vi "test Import To Empty Module Different Slot.vi"(8 "error in (no error)":errorcluster, 11 "TestCase in":refnum<class "SLSC Switch Import Export Unit Tests.lvclass">) -> (0 "error out":errorcluster, 3 "TestCase out":refnum<class "SLSC Switch Import Export Unit Tests.lvclass">)   [LabVIEW 2017, in "SLSC Switch Import Export Unit Tests.lvclass"]
uses:
  SLSC Switch Import Export Unit Tests.lvclass
  Shared/Endpoint Configuration Cluster.ctl
  Shared/Endpoint Configuration Enum.ctl
  SLSC Switch Import Export Unit Tests.lvclass/SLSC Switch Import Export Unit Tests.ctl
  <vilib>/NI Veristand/Custom Device API/Get Item Property (U32).vi
  <vilib>/addons/_JKI Toolkits/VI Tester/TestCase.llb/TestCase.lvclass
  <vilib>/NI/NI VeriStand Custom Device Import and Export Tool/ImportExport.lvlib
  Scripting/SLSC Switch Scripting.lvlib
  Shared/SLSC Switch Shared.lvlib
  <vilib>/NI VeriStand/Custom Device API/Custom Device API.lvlib
  C:/Program Files (x86)/National Instruments/LabVIEW 2017/vi.lib/addons/_JKI Toolkits/VI Tester/TestCase.llb/TestCase.lvclass
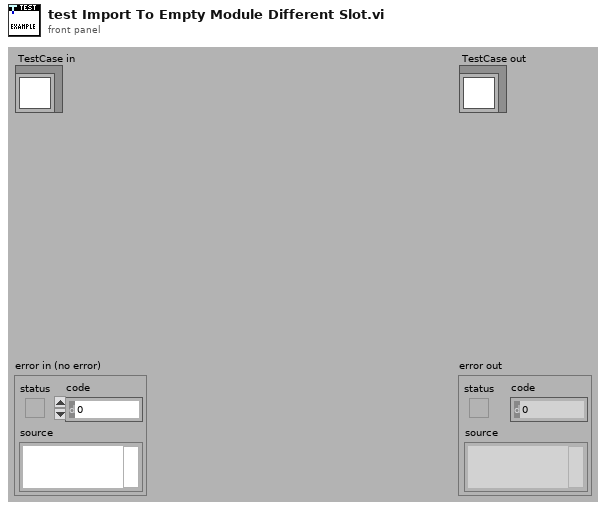
[diagram p1: front panel]
types:
  T1 = cluster{"Ignore Properties":string[], "Ignore Top Level Name":bool}
  T2 = typedef "SLSC Switch Shared.lvlib/Endpoint Configuration Cluster.ctl" = cluster{"Endpoint":string, "Configuration":T3}
  T3 = typedef "SLSC Switch Shared.lvlib/Endpoint Configuration Enum.ctl" = enum16{"Load", "Source", "Configuration"}
  T4 = typedef "Custom Device API.lvlib/Custom Device Item Ref.ctl" = u64
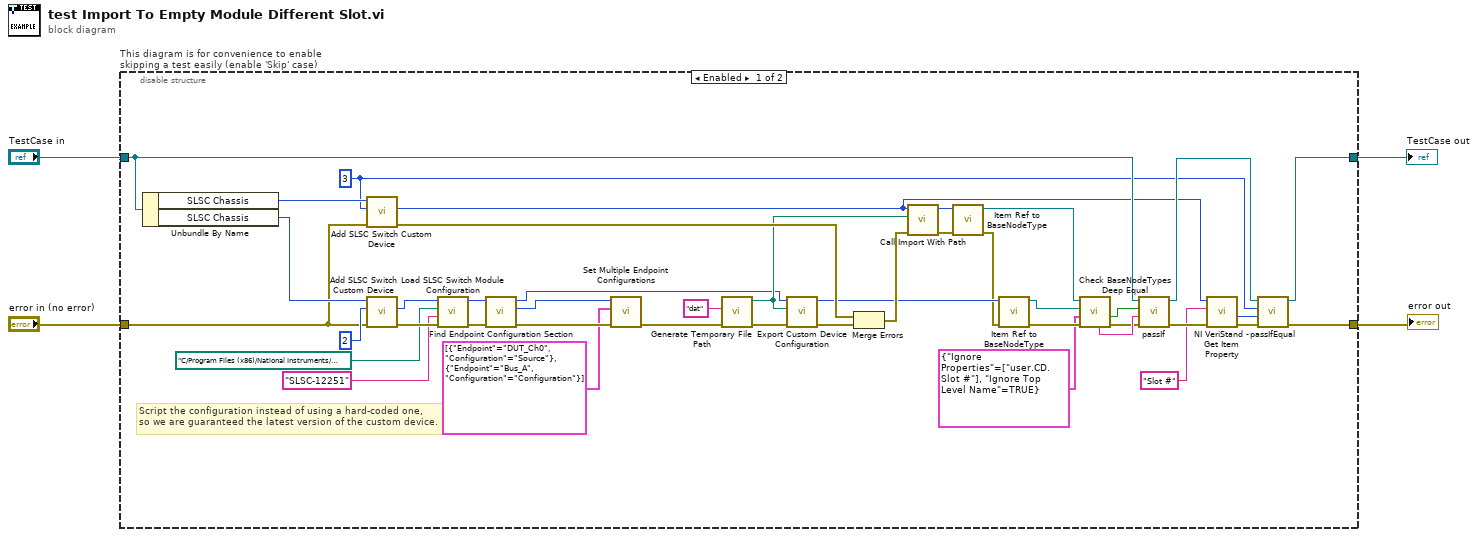
[diagram p0: block diagram]
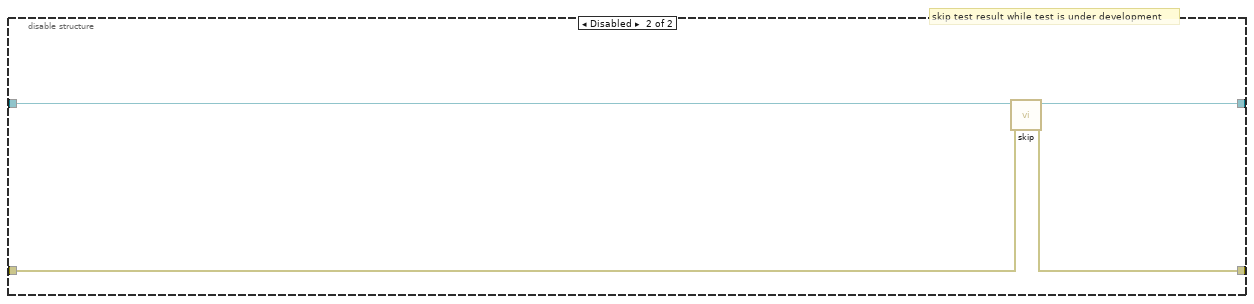
[diagram p2: hidden frame]
diagram:
  n1 = disable-structure "This diagram is for convenience to enable skipping a test easily (enable 'Skip' case)" shown="Enabled" {
    disable-tunnel: "TestCase in" -> [w31 w50]
    disable-tunnel: [w10 w48] -> w1
    disable-tunnel: [w12 w49] -> w3
    disable-tunnel: "error in (no error)" -> [w25 w47]
    frame Enabled {
      w7 = u32 3 ("slot number")
      # "Script the configuration instead of using a hard-coded one,\nso we are guaranteed the latest version of the custom device."
      n2 = Unbundle By Name(w31) -> ("SLSC Chassis"=w26:u64, "SLSC Chassis"=w46:u64)
      n3 = call "Add SLSC Switch Custom Device.vi"("error in"=w25, "slot number"=w7, "slsc chassis in"=w26) -> ("error out"=w41:errorcluster, "slsc switch custom device"=w6:T4)  [unwired: 6 in, 1 out]
      n4 = call "Add SLSC Switch Custom Device.vi"("error in"=w25, "slot number"=u32 2, "slsc chassis in"=w46) -> ("error out"=w24:errorcluster, "slsc switch custom device"=w22:T4)  [unwired: 6 in, 1 out]
      n5 = call "Load SLSC Switch Module Configuration.vi"("error in"=w24, "product name"="SLSC-12251", "switches json file"=path "C:/Program Files (x86)/National Instruments/Shared/NI-SLSC Switch/Modules/SLSC-12251-switches.json", "slsc switch custom device in"=w22) -> ("error out"=w23:errorcluster, "slsc switch custom device out"=w18:T4)  [unwired: 6 in]
      n6 = call "Find Endpoint Configuration Section.vi"("error in"=w23, "slsc switch custom device in"=w18) -> ("error out"=w19:errorcluster, "endpoint configuration"=w16:T4, "slsc switch custom device out"=w15:T4)  [unwired: 7 in]
      n7 = call "Set Multiple Endpoint Configurations.vi"("error in"=w19, "endpoint configurations"=T2[] [{"Endpoint"="DUT_Ch0", "Configuration"=enum."Source"}, {"Endpoint"="Bus_A", "Configuration"=enum."Configuration"}], "endpoint configuration in"=w16) -> ("error out"=w17:errorcluster)  [unwired: 7 in, 1 out]
      n8 = call <vilib>:"Generate Temporary File Path.vi"("error in (no error)"=w17, "Temporary File Extension (tmp)"="dat") -> ("error out"=w43:errorcluster, "Unique Temporary File Path"=w39:path)  [unwired: 8 in]
      n9 = call <vilib>:"Export Custom Device Configuration.vi"("error in (no error)"=w43, "Path"=w39, "ID"=w15) -> ("error out"=w42:errorcluster, "ID out"=w37:u64)  [unwired: 7 in]
      n10 = Merge Errors(w41, w42) -> (w40:errorcluster)
      n11 = call "Call Import With Path.vi"("error in (no error)"=w40, "Path"=w39, "Node Ptr"=w6) -> ("error out"=w36:errorcluster, "Node Ptr out"=w38:u64)  [unwired: 7 in]
      n12 = call "Item Ref to BaseNodeType.vi"("error in (no error)"=w36, "Item Ref"=w38) -> ("error out"=w35:errorcluster, "BaseNodeType"=w28:refnum<k24>)  [unwired: 8 in]
      n13 = call "Item Ref to BaseNodeType.vi"("error in (no error)"=w35, "Item Ref"=w37) -> ("error out"=w34:errorcluster, "BaseNodeType"=w33:refnum<k24>)  [unwired: 8 in]
      n14 = call "Check BaseNodeTypes Deep Equal.vi"("error in (no error)"=w34, "Settings"=T1 {"Ignore Properties"=["user.CD.Slot #"], "Ignore Top Level Name"=TRUE}, "BaseNodeType 2"=w33, "BaseNodeType 1"=w28) -> ("error out"=w27:errorcluster, "Equal?"=w30:bool, "Inequality context"=w29:string)  [unwired: 3 in, 2 out]
      n15 = call-dynamic "passIf.vi"("error in (no error)"=w27, "message (\"\")"=w29, "pass"=w30, "TestCase in"=w31) -> ("error out"=w32:errorcluster, "TestCase out"=w11:refnum<class "SLSC Switch Import Export Unit Tests.lvclass">)  [unwired: 6 in]
      n16 = call-poly <vilib>:"NI VeriStand - Get Item Property.vi"("error in (no error)"=w32, "Property Name"="Slot #", "Item Ref in"=w6) -> ("error out"=w9:errorcluster, "Value"=w8:u32)  [unwired: 5 in, 2 out]
      n17 = call-dynamic "passIfEqual.vi"("error in (no error)"=w9, "y"=w8, "x"=w7, "TestCase in"=w11) -> ("error out"=w12:errorcluster, "TestCase out"=w10:refnum<class "SLSC Switch Import Export Unit Tests.lvclass">)  [unwired: 6 in]
    }
    frame Disabled {
      # "skip test result while test is under development"
      n18 = call <vilib>:"skip.vi"("error in (no error)"=w47, "TestCase in"=w50) -> ("error out"=w49:errorcluster, "TestCase out"=w48:refnum<class "SLSC Switch Import Export Unit Tests.lvclass">)  [unwired: 8 in]
    }
  }
  "error out" <- w3
  "TestCase out" <- w1
